vi "Norland MCA 5500.vi"() -> ()   [LabVIEW 2020]
panel:
  in  "wait time (sec)":dbl=930.0 format="%.2f"
  out "Integral under curve":dbl=2986.0 format="%.2f"
  out "Data":dbl[](array[numeric])=[66.0, 66.0, 79.0, 93.0, 91.0, 111.0, 104.0, 122.0, 123.0, 127.0, 137.0, 132.0, 136.0, 160.0, 142.0, 146.0, 137.0, 117.0, 107.0, 104.0, 103.0, 70.0, 82.0, 61.0, 66.0, 69.0, 49.0, 42.0, 48.0, 47.0, 49.0] format="%.2f"
  out "?":dbl[](graph)
  in  "VISA session":refnum<visa-resource-name>
  in  "End Channel":u32=252
  in  "Start Channel":u32=225
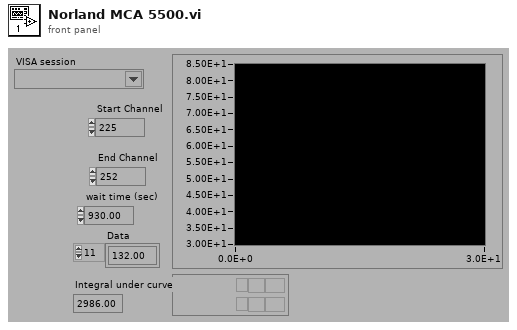
[diagram p1: front panel]
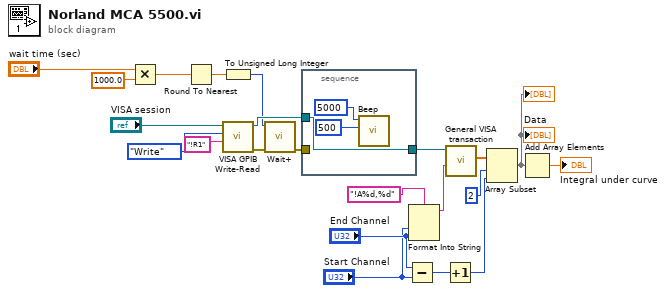
[diagram p0: block diagram]
diagram:
  n1 = Multiply(x="wait time (sec)", y=1000.0) -> (x*y=w17:dbl)
  n2 = Round To Nearest(number=w17) -> (nearest integer value=w2:dbl)
  n3 = To Unsigned Long Integer(number=w2) -> (unsigned 32bit integer=w1:u32)
  n4 = call "VISA GPIB Write-Read.vi"("Command"="!R1", "Action"=enum16{"Write", "Read", "Write & Read"}."Write", "VISA resource name"="VISA session") -> ("error out"=w20:errorcluster, "dup VISA Session"=w4:refnum<visa-resource-name>)  [unwired: 5 in, 2 out]
  n5 = call "Wait+.vi"("Error In"=w20, "milliseconds to wait"=w1) -> ("Error Out"=w3:errorcluster)  [unwired: 4 in, 1 out]
  n6 = stacked-sequence {
    tunnel: w4 -> [w23]
    tunnel: [w23] -> w6
    tunnel: w3 -> [_]
    frame #0 {
      n7 = call <vilib>:"Beep.vi"("duration (msec) - ignored"=500, "frequency (Hz) - ignored"=5000) -> ()  [unwired: 10 in]
    }
  }
  n8 = Subtract(x="End Channel", y="Start Channel") -> (x-y=w12:u32)
  n9 = Format Into String(format string="!A%d,%d", "Start Channel", "End Channel") -> (resulting string=w7:string)  [unwired: 2 in, 1 out]
  n10 = Increment(x=w12) -> (x+1=w11:u32)
  n11 = call "General VISA transaction.vi"("Command String"=w7, "VISA Session"=w6) -> ("Measurement"=w8:dbl[])  [unwired: 4 in, 5 out]
  n12 = Array Subset(array=w8, index=2, length=w11) -> (w10:dbl[])
  "?" <- w10
  "Data" <- w10
  n13 = Add Array Elements(numeric array=w10) -> (sum=→"Integral under curve":dbl)
